vi "configureAnalogOutput.vi"(8 "error in (no error)":errorcluster, 9 "AnalogOutput":refnum<class "AnalogOutput.lvclass">, 10 "deviceName":string, 11 "AtomChipHWC in":refnum<class "AtomChipHWC.lvclass">) -> (0 "error out":errorcluster, 3 "AtomChipHWC out":refnum<class "AtomChipHWC.lvclass">)   [LabVIEW 2011, in "Hardware.lvlib" / "HWControllers.lvlib" / "AtomChipHWC.lvclass"]
doc: "Configure the analog channels of a device"
uses:
  AtomChipHWC.lvclass
  Channels/VoltOutput/AnalogOutput.lvclass
  AtomChipHWC.lvclass/AtomChipHWC.ctl
  HWController.lvclass
  Tools/Filing/FileNeologist/FileNeologist.lvclass
  Tools/Filing.lvlib
  Tools/DatabaseHelpers/DbConnection/DeviceDataBase/deviceDataBase.lvclass
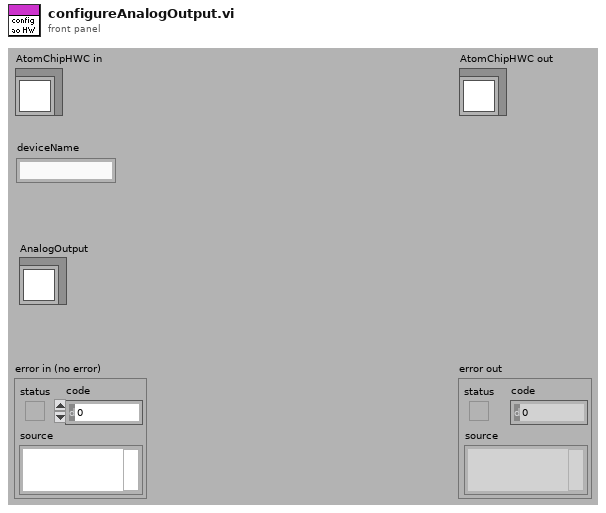
[diagram p1: front panel]
types:
  T1 = cluster{string, "Physical Channels":string, "Ranges":dbl[]}
  T2 = cluster{"Clock source":string, "Clock rate":dbl, "Start trigger line":string, "Sample Rate":dbl, "Sample No.":dbl}
  T3 = cluster{"Range":cluster{"current":dbl, "voltage":dbl}, "triggering_inUse":cluster{"start_trigger":string, "clock":string}, "Limits":cluster{"VoltageLimit":dbl, "CurrentLimit":dbl}}[]
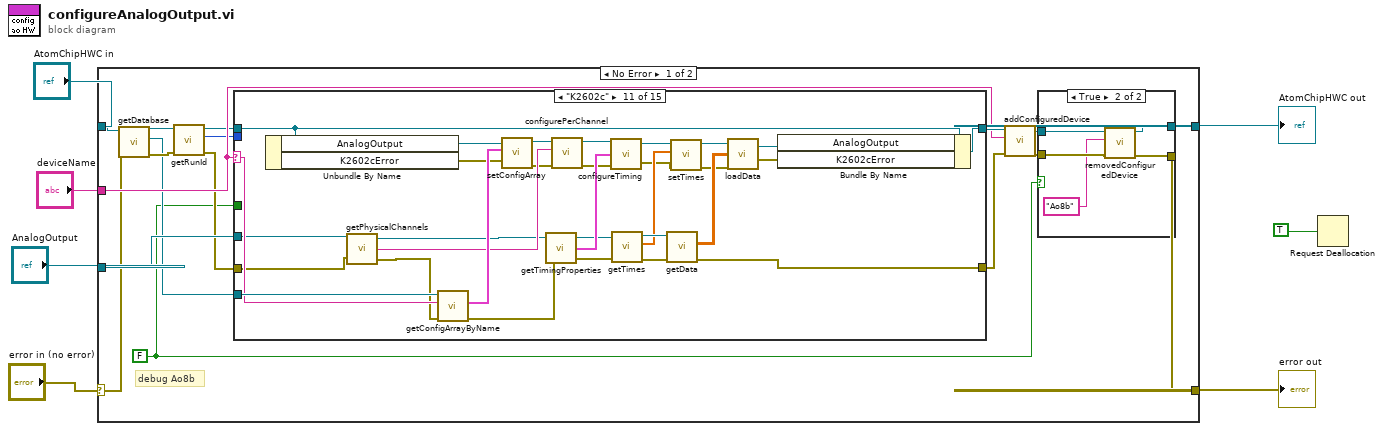
[diagram p0: block diagram]
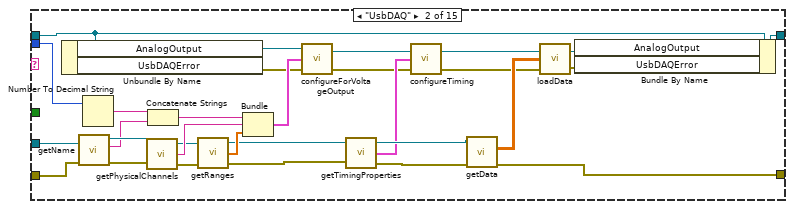
[diagram p4: hidden frame]
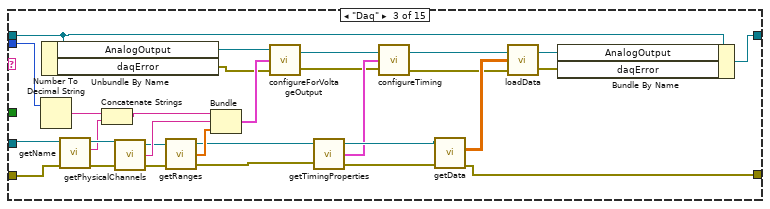
[diagram p5: hidden frame]
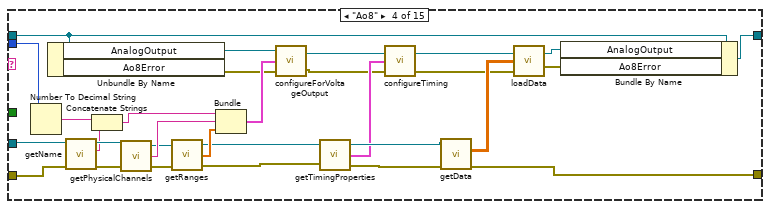
[diagram p6: hidden frame]
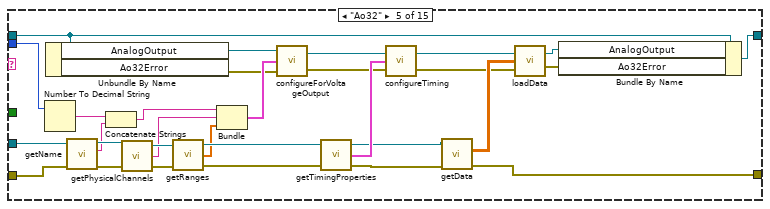
[diagram p7: hidden frame]
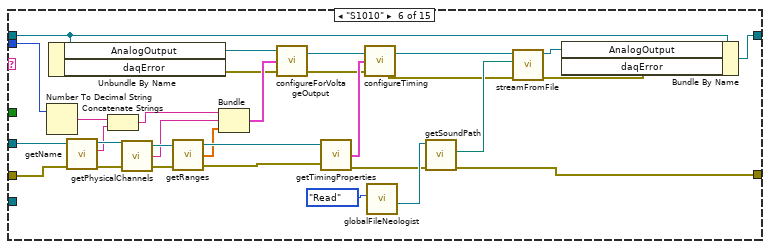
[diagram p8: hidden frame]
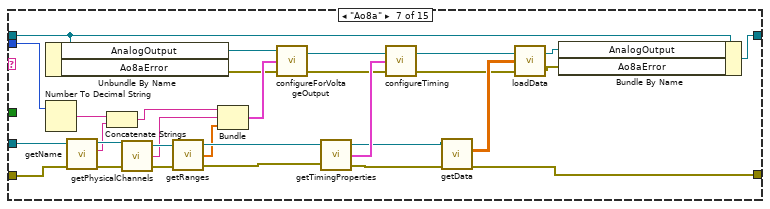
[diagram p9: hidden frame]
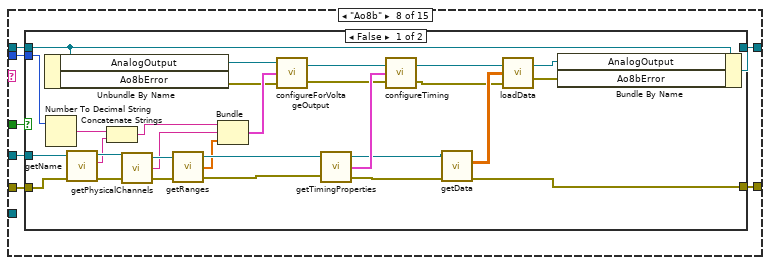
[diagram p10: hidden frame]
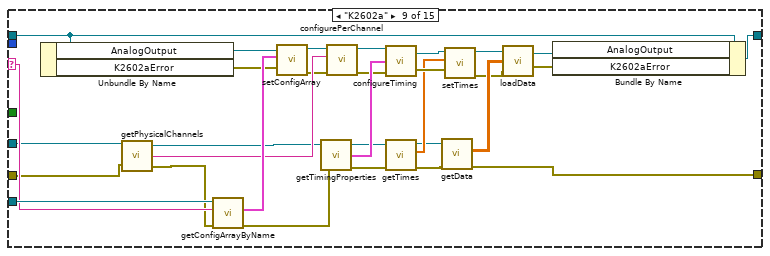
[diagram p12: hidden frame]
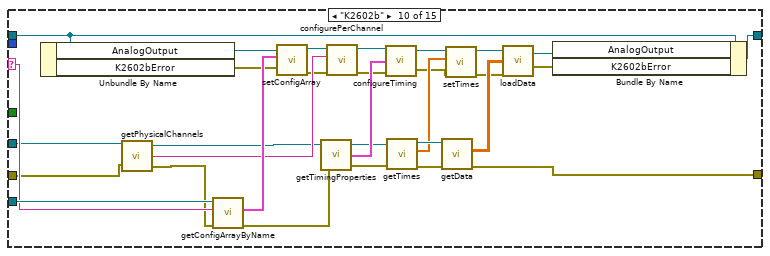
[diagram p13: hidden frame]
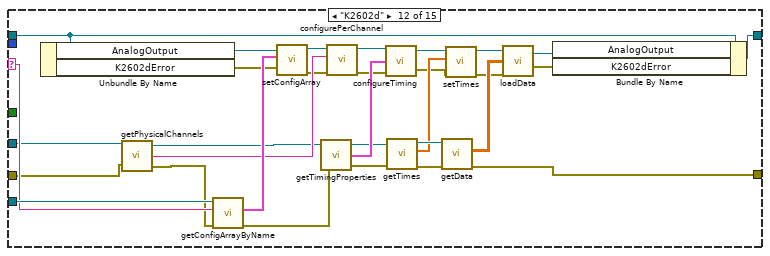
[diagram p14: hidden frame]
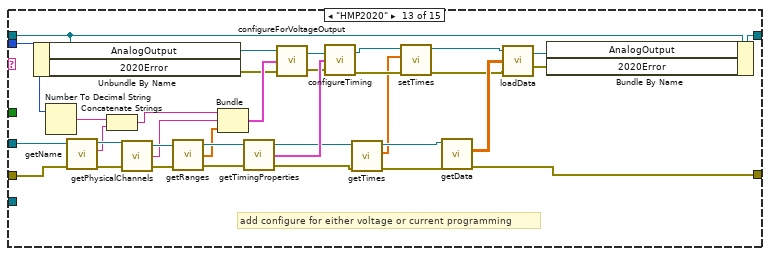
[diagram p15: hidden frame]
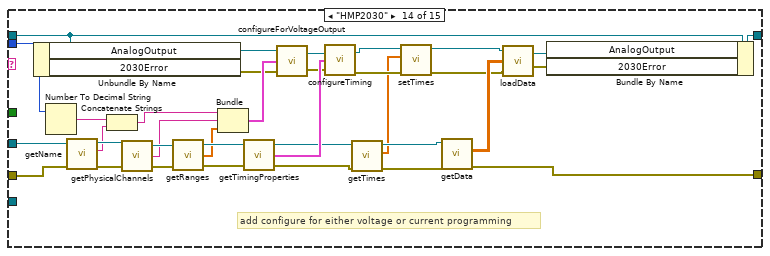
[diagram p16: hidden frame]
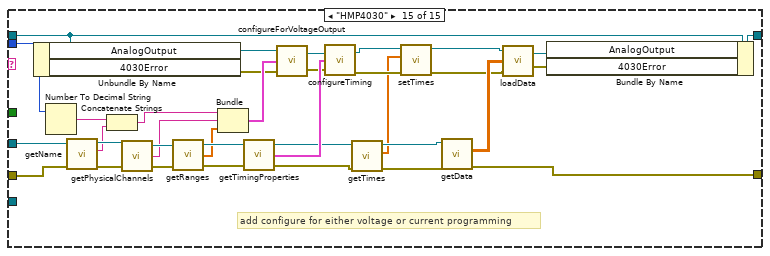
[diagram p17: hidden frame]
diagram:
  n1 = case shown="No Error" "error in (no error)" {
    selector: "error in (no error)" -> [w15 w484]
    tunnel: [w9 w484] -> w6
    tunnel: [w11 w483] -> w4
    tunnel: "AtomChipHWC in" -> [w16 w483]
    tunnel: "deviceName" -> [w21 _]
    tunnel: "AnalogOutput" -> [w24 _]
    frame No Error {
      w8 = FALSE
      # "debug Ao8b"
      n2 = call "getDatabase.vi"("error in (no error)"=w15, "HWController in"=w16) -> ("error out"=w14:errorcluster, "deviceDataBase"=w13:refnum<class "deviceDataBase.lvclass">, "HWController out"=w17:refnum<class "AtomChipHWC.lvclass">)  [unwired: 7 in]
      n3 = call "getRunId.vi"("error in (no error)"=w14, "HWController in"=w17) -> ("error out"=w19:errorcluster, "Numeric"=w18:i32, "HWController out"=w20:refnum<class "AtomChipHWC.lvclass">)  [unwired: 7 in]
      n4 = case shown="\"K2602c\"" w21 {
        selector: w21 -> [_ _ _ _ _ _ _ _ w276 w307 w338 w369 _ _ _]
        tunnel: w20 -> [w33 w48 w78 w108 w153 w184 w214 w221 w284 w315 w346 w377 w412 w447 w482]
        tunnel: [w33 w47 w77 w107 w152 w183 w213 w220 w283 w314 w345 w376 w411 w446 w481] -> w23
        tunnel: [w32 w34 w65 w95 w126 w156 w185 w216 w278 w309 w340 w371 w388 w423 w458] -> w22
        tunnel: w24 -> [_ w46 w76 w106 w145 w176 w206 w218 w270 w301 w332 w363 w404 w439 w474]
        tunnel: w19 -> [w32 w45 w75 w105 w146 w177 w207 w219 w269 w300 w331 w362 w405 w440 w475]
        tunnel: w18 -> [_ w41 w73 w103 w133 w168 w194 w217 _ _ _ _ w394 w429 w464]
        tunnel: w13 -> [_ _ _ _ _ _ _ _ w277 w308 w339 w370 _ _ _]
        tunnel: w8 -> [_ _ _ _ _ _ _ w215 _ _ _ _ _ _ _]
        frame "No Hardware", Default {
        }
        frame "UsbDAQ" {
          n5 = Unbundle By Name(w48) -> ("AnalogOutput"=w54:refnum<class "AnalogOutput.lvclass">, "UsbDAQError"=w37:errorcluster)
          n6 = call "getName.vi"("error in (no error)"=w45, "AnalogOutput.lvclass in"=w46) -> ("error out"=w49:errorcluster, "name"=w43:string, "AnalogOutput.lvclass out"=w51:refnum<class "AnalogOutput.lvclass">)  [unwired: 7 in]
          n7 = Number To Decimal String(number=w41) -> (decimal integer string=w44:string)  [unwired: 1 in]
          n8 = call-dynamic "getPhysicalChannels.vi"("AnalogOutput.lvclass in"=w51, "error in (no error)"=w49) -> ("AnalogOutput.lvclass out"=w52:refnum<class "AnalogOutput.lvclass">, "Physical Channels"=w55:string, "error out"=w50:errorcluster)
          n9 = Concatenate Strings(w44, w43) -> (w42:string)
          n10 = call "getRanges.vi"("AnalogOutput.lvclass in"=w52, "error in (no error)"=w50) -> ("AnalogOutput.lvclass out"=w53:refnum<class "AnalogOutput.lvclass">, "Ranges"=w56:dbl[], "error out"=w36:errorcluster)
          n11 = Bundle(w42, "Physical Channels"=w55, "Ranges"=w56) -> (w57:T1)  [unwired: 1 in]
          n12 = call-dynamic "configureForVoltageOutput.vi"("error in (no error)"=w37, "Output Properties"=w57, "AnalogOutput in"=w54) -> ("error out"=w38:errorcluster, "AnalogOutput out"=w60:refnum<class "AnalogOutput.lvclass">)
          n13 = call "getTimingProperties.vi"("AnalogOutput.lvclass in"=w53, "error in (no error)"=w36) -> ("AnalogOutput.lvclass out"=w59:refnum<class "AnalogOutput.lvclass">, "Timing"=w58:T2, "error out"=w35:errorcluster)
          n14 = call-dynamic "configureTiming.vi"("error in (no error)"=w38, "Timing"=w58, "AnalogOutput in"=w60) -> ("error out"=w39:errorcluster, "AnalogOutput out"=w61:refnum<class "AnalogOutput.lvclass">)
          n15 = call "getData.vi"("error in (no error)"=w35, "AnalogOutput.lvclass in"=w59) -> ("error out"=w34:errorcluster, "Data"=w62:dbl[][])  [unwired: 7 in, 1 out]
          n16 = call-dynamic "loadData.vi"("error in (no error)"=w39, "Data"=w62, "AnalogOutput in"=w61) -> ("error out"=w40:errorcluster, "AnalogOutput out"=w63:refnum<class "AnalogOutput.lvclass">)
          n17 = Bundle By Name(cluster=w48, "AnalogOutput"=w63, "UsbDAQError"=w40) -> (w47:refnum<class "AtomChipHWC.lvclass">)
        }
        frame "Daq" {
          n18 = Number To Decimal String(number=w73) -> (decimal integer string=w74:string)  [unwired: 1 in]
          n19 = Unbundle By Name(w78) -> ("AnalogOutput"=w84:refnum<class "AnalogOutput.lvclass">, "daqError"=w68:errorcluster)
          n20 = call "getName.vi"("error in (no error)"=w75, "AnalogOutput.lvclass in"=w76) -> ("error out"=w79:errorcluster, "name"=w72:string, "AnalogOutput.lvclass out"=w81:refnum<class "AnalogOutput.lvclass">)  [unwired: 7 in]
          n21 = Concatenate Strings(w74, w72) -> (w71:string)
          n22 = call-dynamic "getPhysicalChannels.vi"("AnalogOutput.lvclass in"=w81, "error in (no error)"=w79) -> ("AnalogOutput.lvclass out"=w82:refnum<class "AnalogOutput.lvclass">, "Physical Channels"=w85:string, "error out"=w80:errorcluster)
          n23 = call "getRanges.vi"("AnalogOutput.lvclass in"=w82, "error in (no error)"=w80) -> ("AnalogOutput.lvclass out"=w83:refnum<class "AnalogOutput.lvclass">, "Ranges"=w86:dbl[], "error out"=w70:errorcluster)
          n24 = Bundle(w71, "Physical Channels"=w85, "Ranges"=w86) -> (w87:T1)  [unwired: 1 in]
          n25 = call-dynamic "configureForVoltageOutput.vi"("error in (no error)"=w68, "Output Properties"=w87, "AnalogOutput in"=w84) -> ("error out"=w66:errorcluster, "AnalogOutput out"=w90:refnum<class "AnalogOutput.lvclass">)
          n26 = call "getTimingProperties.vi"("AnalogOutput.lvclass in"=w83, "error in (no error)"=w70) -> ("AnalogOutput.lvclass out"=w89:refnum<class "AnalogOutput.lvclass">, "Timing"=w88:T2, "error out"=w67:errorcluster)
          n27 = call-dynamic "configureTiming.vi"("error in (no error)"=w66, "Timing"=w88, "AnalogOutput in"=w90) -> ("error out"=w69:errorcluster, "AnalogOutput out"=w91:refnum<class "AnalogOutput.lvclass">)
          n28 = call "getData.vi"("error in (no error)"=w67, "AnalogOutput.lvclass in"=w89) -> ("error out"=w65:errorcluster, "Data"=w92:dbl[][])  [unwired: 7 in, 1 out]
          n29 = call-dynamic "loadData.vi"("error in (no error)"=w69, "Data"=w92, "AnalogOutput in"=w91) -> ("error out"=w64:errorcluster, "AnalogOutput out"=w93:refnum<class "AnalogOutput.lvclass">)
          n30 = Bundle By Name(cluster=w78, "AnalogOutput"=w93, "daqError"=w64) -> (w77:refnum<class "AtomChipHWC.lvclass">)
        }
        frame "Ao8" {
          n31 = Number To Decimal String(number=w103) -> (decimal integer string=w104:string)  [unwired: 1 in]
          n32 = Unbundle By Name(w108) -> ("AnalogOutput"=w114:refnum<class "AnalogOutput.lvclass">, "Ao8Error"=w98:errorcluster)
          n33 = call "getName.vi"("error in (no error)"=w105, "AnalogOutput.lvclass in"=w106) -> ("error out"=w109:errorcluster, "name"=w102:string, "AnalogOutput.lvclass out"=w111:refnum<class "AnalogOutput.lvclass">)  [unwired: 7 in]
          n34 = Concatenate Strings(w104, w102) -> (w101:string)
          n35 = call-dynamic "getPhysicalChannels.vi"("AnalogOutput.lvclass in"=w111, "error in (no error)"=w109) -> ("AnalogOutput.lvclass out"=w112:refnum<class "AnalogOutput.lvclass">, "Physical Channels"=w115:string, "error out"=w110:errorcluster)
          n36 = call "getRanges.vi"("AnalogOutput.lvclass in"=w112, "error in (no error)"=w110) -> ("AnalogOutput.lvclass out"=w113:refnum<class "AnalogOutput.lvclass">, "Ranges"=w116:dbl[], "error out"=w97:errorcluster)
          n37 = Bundle(w101, "Physical Channels"=w115, "Ranges"=w116) -> (w117:T1)  [unwired: 1 in]
          n38 = call-dynamic "configureForVoltageOutput.vi"("error in (no error)"=w98, "Output Properties"=w117, "AnalogOutput in"=w114) -> ("error out"=w99:errorcluster, "AnalogOutput out"=w120:refnum<class "AnalogOutput.lvclass">)
          n39 = call "getTimingProperties.vi"("AnalogOutput.lvclass in"=w113, "error in (no error)"=w97) -> ("AnalogOutput.lvclass out"=w119:refnum<class "AnalogOutput.lvclass">, "Timing"=w118:T2, "error out"=w96:errorcluster)
          n40 = call-dynamic "configureTiming.vi"("error in (no error)"=w99, "Timing"=w118, "AnalogOutput in"=w120) -> ("error out"=w100:errorcluster, "AnalogOutput out"=w121:refnum<class "AnalogOutput.lvclass">)
          n41 = call "getData.vi"("error in (no error)"=w96, "AnalogOutput.lvclass in"=w119) -> ("error out"=w95:errorcluster, "Data"=w122:dbl[][])  [unwired: 7 in, 1 out]
          n42 = call-dynamic "loadData.vi"("error in (no error)"=w100, "Data"=w122, "AnalogOutput in"=w121) -> ("error out"=w94:errorcluster, "AnalogOutput out"=w123:refnum<class "AnalogOutput.lvclass">)
          n43 = Bundle By Name(cluster=w108, "AnalogOutput"=w123, "Ao8Error"=w94) -> (w107:refnum<class "AtomChipHWC.lvclass">)
        }
        frame "Ao32" {
          n44 = Number To Decimal String(number=w133) -> (decimal integer string=w134:string)  [unwired: 1 in]
          n45 = Unbundle By Name(w153) -> ("AnalogOutput"=w144:refnum<class "AnalogOutput.lvclass">, "Ao32Error"=w130:errorcluster)
          n46 = call "getName.vi"("error in (no error)"=w146, "AnalogOutput.lvclass in"=w145) -> ("error out"=w151:errorcluster, "name"=w132:string, "AnalogOutput.lvclass out"=w149:refnum<class "AnalogOutput.lvclass">)  [unwired: 7 in]
          n47 = Concatenate Strings(w134, w132) -> (w131:string)
          n48 = call-dynamic "getPhysicalChannels.vi"("AnalogOutput.lvclass in"=w149, "error in (no error)"=w151) -> ("AnalogOutput.lvclass out"=w148:refnum<class "AnalogOutput.lvclass">, "Physical Channels"=w143:string, "error out"=w150:errorcluster)
          n49 = call "getRanges.vi"("AnalogOutput.lvclass in"=w148, "error in (no error)"=w150) -> ("AnalogOutput.lvclass out"=w147:refnum<class "AnalogOutput.lvclass">, "Ranges"=w142:dbl[], "error out"=w124:errorcluster)
          n50 = Bundle(w131, "Physical Channels"=w143, "Ranges"=w142) -> (w141:T1)  [unwired: 1 in]
          n51 = call-dynamic "configureForVoltageOutput.vi"("error in (no error)"=w130, "Output Properties"=w141, "AnalogOutput in"=w144) -> ("error out"=w129:errorcluster, "AnalogOutput out"=w138:refnum<class "AnalogOutput.lvclass">)
          n52 = call "getTimingProperties.vi"("AnalogOutput.lvclass in"=w147, "error in (no error)"=w124) -> ("AnalogOutput.lvclass out"=w139:refnum<class "AnalogOutput.lvclass">, "Timing"=w140:T2, "error out"=w125:errorcluster)
          n53 = call-dynamic "configureTiming.vi"("error in (no error)"=w129, "Timing"=w140, "AnalogOutput in"=w138) -> ("error out"=w128:errorcluster, "AnalogOutput out"=w137:refnum<class "AnalogOutput.lvclass">)
          n54 = call "getData.vi"("error in (no error)"=w125, "AnalogOutput.lvclass in"=w139) -> ("error out"=w126:errorcluster, "Data"=w136:dbl[][])  [unwired: 7 in, 1 out]
          n55 = call-dynamic "loadData.vi"("error in (no error)"=w128, "Data"=w136, "AnalogOutput in"=w137) -> ("error out"=w127:errorcluster, "AnalogOutput out"=w135:refnum<class "AnalogOutput.lvclass">)
          n56 = Bundle By Name(cluster=w153, "AnalogOutput"=w135, "Ao32Error"=w127) -> (w152:refnum<class "AtomChipHWC.lvclass">)
        }
        frame "S1010" {
          n57 = Number To Decimal String(number=w168) -> (decimal integer string=w169:string)  [unwired: 1 in]
          n58 = Unbundle By Name(w184) -> ("AnalogOutput"=w175:refnum<class "AnalogOutput.lvclass">, "daqError"=w158:errorcluster)
          n59 = call "getName.vi"("error in (no error)"=w177, "AnalogOutput.lvclass in"=w176) -> ("error out"=w182:errorcluster, "name"=w167:string, "AnalogOutput.lvclass out"=w180:refnum<class "AnalogOutput.lvclass">)  [unwired: 7 in]
          n60 = Concatenate Strings(w169, w167) -> (w166:string)
          n61 = call-dynamic "getPhysicalChannels.vi"("AnalogOutput.lvclass in"=w180, "error in (no error)"=w182) -> ("AnalogOutput.lvclass out"=w179:refnum<class "AnalogOutput.lvclass">, "Physical Channels"=w174:string, "error out"=w181:errorcluster)
          n62 = call "getRanges.vi"("AnalogOutput.lvclass in"=w179, "error in (no error)"=w181) -> ("AnalogOutput.lvclass out"=w178:refnum<class "AnalogOutput.lvclass">, "Ranges"=w173:dbl[], "error out"=w154:errorcluster)
          n63 = Bundle(w166, "Physical Channels"=w174, "Ranges"=w173) -> (w172:T1)  [unwired: 1 in]
          n64 = call-dynamic "configureForVoltageOutput.vi"("error in (no error)"=w158, "Output Properties"=w172, "AnalogOutput in"=w175) -> ("error out"=w159:errorcluster, "AnalogOutput out"=w170:refnum<class "AnalogOutput.lvclass">)
          n65 = call "getTimingProperties.vi"("AnalogOutput.lvclass in"=w178, "error in (no error)"=w154) -> ("Timing"=w171:T2, "error out"=w155:errorcluster)  [unwired: 1 out]
          n66 = call-dynamic "configureTiming.vi"("error in (no error)"=w159, "Timing"=w171, "AnalogOutput in"=w170) -> ("error out"=w160:errorcluster, "AnalogOutput out"=w165:refnum<class "AnalogOutput.lvclass">)
          n67 = call "globalFileNeologist.vi"("Action"=enum16{"Write", "Read"}."Read") -> ("FileNeologist out"=w163:refnum<class "FileNeologist.lvclass">)  [unwired: 10 in]
          n68 = call "getSoundPath.vi"("error in (no error)"=w155, "FileNeologist in"=w163) -> ("error out"=w156:errorcluster, "Path"=w161:path)  [unwired: 7 in, 1 out]
          n69 = call-dynamic "streamFromFile.vi"("error in (no error)"=w160, "Path"=w161, "AnalogOutput in"=w165) -> ("error out"=w157:errorcluster, "AnalogOutput out"=w164:refnum<class "AnalogOutput.lvclass">)  [unwired: 7 in]
          n70 = Bundle By Name(cluster=w184, "AnalogOutput"=w164, "daqError"=w157) -> (w183:refnum<class "AtomChipHWC.lvclass">)
        }
        frame "Ao8a" {
          n71 = Unbundle By Name(w214) -> ("AnalogOutput"=w205:refnum<class "AnalogOutput.lvclass">, "Ao8aError"=w189:errorcluster)
          n72 = Number To Decimal String(number=w194) -> (decimal integer string=w195:string)  [unwired: 1 in]
          n73 = call "getName.vi"("error in (no error)"=w207, "AnalogOutput.lvclass in"=w206) -> ("error out"=w212:errorcluster, "name"=w193:string, "AnalogOutput.lvclass out"=w210:refnum<class "AnalogOutput.lvclass">)  [unwired: 7 in]
          n74 = Concatenate Strings(w195, w193) -> (w192:string)
          n75 = call-dynamic "getPhysicalChannels.vi"("AnalogOutput.lvclass in"=w210, "error in (no error)"=w212) -> ("AnalogOutput.lvclass out"=w209:refnum<class "AnalogOutput.lvclass">, "Physical Channels"=w204:string, "error out"=w211:errorcluster)
          n76 = call "getRanges.vi"("AnalogOutput.lvclass in"=w209, "error in (no error)"=w211) -> ("AnalogOutput.lvclass out"=w208:refnum<class "AnalogOutput.lvclass">, "Ranges"=w203:dbl[], "error out"=w186:errorcluster)
          n77 = Bundle(w192, "Physical Channels"=w204, "Ranges"=w203) -> (w202:T1)  [unwired: 1 in]
          n78 = call-dynamic "configureForVoltageOutput.vi"("error in (no error)"=w189, "Output Properties"=w202, "AnalogOutput in"=w205) -> ("error out"=w190:errorcluster, "AnalogOutput out"=w199:refnum<class "AnalogOutput.lvclass">)
          n79 = call "getTimingProperties.vi"("AnalogOutput.lvclass in"=w208, "error in (no error)"=w186) -> ("AnalogOutput.lvclass out"=w200:refnum<class "AnalogOutput.lvclass">, "Timing"=w201:T2, "error out"=w187:errorcluster)
          n80 = call-dynamic "configureTiming.vi"("error in (no error)"=w190, "Timing"=w201, "AnalogOutput in"=w199) -> ("error out"=w191:errorcluster, "AnalogOutput out"=w198:refnum<class "AnalogOutput.lvclass">)
          n81 = call "getData.vi"("error in (no error)"=w187, "AnalogOutput.lvclass in"=w200) -> ("error out"=w185:errorcluster, "Data"=w197:dbl[][])  [unwired: 7 in, 1 out]
          n82 = call-dynamic "loadData.vi"("error in (no error)"=w191, "Data"=w197, "AnalogOutput in"=w198) -> ("error out"=w188:errorcluster, "AnalogOutput out"=w196:refnum<class "AnalogOutput.lvclass">)
          n83 = Bundle By Name(cluster=w214, "AnalogOutput"=w196, "Ao8aError"=w188) -> (w213:refnum<class "AtomChipHWC.lvclass">)
        }
        frame "Ao8b" {
          n84 = case shown="False" w215 {
            tunnel: w221 -> [w251 w253]
            tunnel: [w250 w253] -> w220
            tunnel: w219 -> [w249 w252]
            tunnel: w218 -> [w248 _]
            tunnel: w217 -> [w247 _]
            tunnel: [w246 w252] -> w216
            frame False {
              n85 = Unbundle By Name(w251) -> ("AnalogOutput"=w240:refnum<class "AnalogOutput.lvclass">, "Ao8bError"=w227:errorcluster)
              n86 = Number To Decimal String(number=w247) -> (decimal integer string=w230:string)  [unwired: 1 in]
              n87 = call "getName.vi"("error in (no error)"=w249, "AnalogOutput.lvclass in"=w248) -> ("error out"=w245:errorcluster, "name"=w229:string, "AnalogOutput.lvclass out"=w243:refnum<class "AnalogOutput.lvclass">)  [unwired: 7 in]
              n88 = Concatenate Strings(w230, w229) -> (w228:string)
              n89 = call-dynamic "getPhysicalChannels.vi"("AnalogOutput.lvclass in"=w243, "error in (no error)"=w245) -> ("AnalogOutput.lvclass out"=w242:refnum<class "AnalogOutput.lvclass">, "Physical Channels"=w239:string, "error out"=w244:errorcluster)
              n90 = call "getRanges.vi"("AnalogOutput.lvclass in"=w242, "error in (no error)"=w244) -> ("AnalogOutput.lvclass out"=w241:refnum<class "AnalogOutput.lvclass">, "Ranges"=w238:dbl[], "error out"=w222:errorcluster)
              n91 = Bundle(w228, "Physical Channels"=w239, "Ranges"=w238) -> (w237:T1)  [unwired: 1 in]
              n92 = call-dynamic "configureForVoltageOutput.vi"("error in (no error)"=w227, "Output Properties"=w237, "AnalogOutput in"=w240) -> ("error out"=w226:errorcluster, "AnalogOutput out"=w234:refnum<class "AnalogOutput.lvclass">)
              n93 = call "getTimingProperties.vi"("AnalogOutput.lvclass in"=w241, "error in (no error)"=w222) -> ("AnalogOutput.lvclass out"=w235:refnum<class "AnalogOutput.lvclass">, "Timing"=w236:T2, "error out"=w223:errorcluster)
              n94 = call-dynamic "configureTiming.vi"("error in (no error)"=w226, "Timing"=w236, "AnalogOutput in"=w234) -> ("error out"=w225:errorcluster, "AnalogOutput out"=w233:refnum<class "AnalogOutput.lvclass">)
              n95 = call "getData.vi"("error in (no error)"=w223, "AnalogOutput.lvclass in"=w235) -> ("error out"=w246:errorcluster, "Data"=w232:dbl[][])  [unwired: 7 in, 1 out]
              n96 = call-dynamic "loadData.vi"("error in (no error)"=w225, "Data"=w232, "AnalogOutput in"=w233) -> ("error out"=w224:errorcluster, "AnalogOutput out"=w231:refnum<class "AnalogOutput.lvclass">)
              n97 = Bundle By Name(cluster=w251, "AnalogOutput"=w231, "Ao8bError"=w224) -> (w250:refnum<class "AtomChipHWC.lvclass">)
            }
            frame True {
            }
          }
        }
        frame "K2602a" {
          n98 = Unbundle By Name(w284) -> ("AnalogOutput"=w266:refnum<class "AnalogOutput.lvclass">, "K2602aError"=w263:errorcluster)
          n99 = call-dynamic "getPhysicalChannels.vi"("AnalogOutput.lvclass in"=w270, "error in (no error)"=w269) -> ("AnalogOutput.lvclass out"=w272:refnum<class "AnalogOutput.lvclass">, "Physical Channels"=w273:string, "error out"=w271:errorcluster)
          n100 = call "getConfigArrayByName.vi"("error in (no error)"=w271, "device_name"=w276, "deviceDataBase in"=w277) -> ("error out"=w275:errorcluster, "ConfigArray"=w274:T3)  [unwired: 6 in, 1 out]
          n101 = call-dynamic "setConfigArray.vi"("error in (no error)"=w263, "ConfigArray"=w274, "AnalogOutput in"=w266) -> ("error out"=w264:errorcluster, "AnalogOutput out"=w265:refnum<class "AnalogOutput.lvclass">)  [unwired: 7 in]
          n102 = call "getTimingProperties.vi"("AnalogOutput.lvclass in"=w272, "error in (no error)"=w275) -> ("AnalogOutput.lvclass out"=w258:refnum<class "AnalogOutput.lvclass">, "Timing"=w282:T2, "error out"=w257:errorcluster)
          n103 = call-dynamic "configurePerChannel.vi"("error in (no error)"=w264, "physical channels"=w273, "AnalogOutput in"=w265) -> ("error out"=w267:errorcluster, "AnalogOutput out"=w268:refnum<class "AnalogOutput.lvclass">)  [unwired: 7 in]
          n104 = call-dynamic "configureTiming.vi"("error in (no error)"=w267, "Timing"=w282, "AnalogOutput in"=w268) -> ("error out"=w261:errorcluster, "AnalogOutput out"=w262:refnum<class "AnalogOutput.lvclass">)
          n105 = call "getTimes.vi"("error in (no error)"=w257, "AnalogOutput in"=w258) -> ("error out"=w256:errorcluster, "times"=w255:dbl[], "AnalogOutput out"=w254:refnum<class "AnalogOutput.lvclass">)  [unwired: 7 in]
          n106 = call "getData.vi"("error in (no error)"=w256, "AnalogOutput.lvclass in"=w254) -> ("error out"=w278:errorcluster, "Data"=w281:dbl[][])  [unwired: 7 in, 1 out]
          n107 = call "setTimes.vi"("error in (no error)"=w261, "times"=w255, "AnalogOutput in"=w262) -> ("error out"=w260:errorcluster, "AnalogOutput out"=w259:refnum<class "AnalogOutput.lvclass">)  [unwired: 7 in]
          n108 = call-dynamic "loadData.vi"("error in (no error)"=w260, "Data"=w281, "AnalogOutput in"=w259) -> ("error out"=w279:errorcluster, "AnalogOutput out"=w280:refnum<class "AnalogOutput.lvclass">)
          n109 = Bundle By Name(cluster=w284, "AnalogOutput"=w280, "K2602aError"=w279) -> (w283:refnum<class "AtomChipHWC.lvclass">)
        }
        frame "K2602b" {
          n110 = Unbundle By Name(w315) -> ("AnalogOutput"=w297:refnum<class "AnalogOutput.lvclass">, "K2602bError"=w294:errorcluster)
          n111 = call-dynamic "getPhysicalChannels.vi"("AnalogOutput.lvclass in"=w301, "error in (no error)"=w300) -> ("AnalogOutput.lvclass out"=w303:refnum<class "AnalogOutput.lvclass">, "Physical Channels"=w304:string, "error out"=w302:errorcluster)
          n112 = call "getConfigArrayByName.vi"("error in (no error)"=w302, "device_name"=w307, "deviceDataBase in"=w308) -> ("error out"=w306:errorcluster, "ConfigArray"=w305:T3)  [unwired: 6 in, 1 out]
          n113 = call-dynamic "setConfigArray.vi"("error in (no error)"=w294, "ConfigArray"=w305, "AnalogOutput in"=w297) -> ("error out"=w295:errorcluster, "AnalogOutput out"=w296:refnum<class "AnalogOutput.lvclass">)  [unwired: 7 in]
          n114 = call "getTimingProperties.vi"("AnalogOutput.lvclass in"=w303, "error in (no error)"=w306) -> ("AnalogOutput.lvclass out"=w293:refnum<class "AnalogOutput.lvclass">, "Timing"=w313:T2, "error out"=w285:errorcluster)
          n115 = call-dynamic "configurePerChannel.vi"("error in (no error)"=w295, "physical channels"=w304, "AnalogOutput in"=w296) -> ("error out"=w298:errorcluster, "AnalogOutput out"=w299:refnum<class "AnalogOutput.lvclass">)  [unwired: 7 in]
          n116 = call-dynamic "configureTiming.vi"("error in (no error)"=w298, "Timing"=w313, "AnalogOutput in"=w299) -> ("error out"=w289:errorcluster, "AnalogOutput out"=w290:refnum<class "AnalogOutput.lvclass">)
          n117 = call "getTimes.vi"("error in (no error)"=w285, "AnalogOutput in"=w293) -> ("error out"=w286:errorcluster, "times"=w291:dbl[], "AnalogOutput out"=w292:refnum<class "AnalogOutput.lvclass">)  [unwired: 7 in]
          n118 = call "getData.vi"("error in (no error)"=w286, "AnalogOutput.lvclass in"=w292) -> ("error out"=w309:errorcluster, "Data"=w312:dbl[][])  [unwired: 7 in, 1 out]
          n119 = call "setTimes.vi"("error in (no error)"=w289, "times"=w291, "AnalogOutput in"=w290) -> ("error out"=w288:errorcluster, "AnalogOutput out"=w287:refnum<class "AnalogOutput.lvclass">)  [unwired: 7 in]
          n120 = call-dynamic "loadData.vi"("error in (no error)"=w288, "Data"=w312, "AnalogOutput in"=w287) -> ("error out"=w310:errorcluster, "AnalogOutput out"=w311:refnum<class "AnalogOutput.lvclass">)
          n121 = Bundle By Name(cluster=w315, "AnalogOutput"=w311, "K2602bError"=w310) -> (w314:refnum<class "AtomChipHWC.lvclass">)
        }
        frame "K2602c" {
          n122 = Unbundle By Name(w346) -> ("AnalogOutput"=w328:refnum<class "AnalogOutput.lvclass">, "K2602cError"=w325:errorcluster)
          n123 = call-dynamic "getPhysicalChannels.vi"("AnalogOutput.lvclass in"=w332, "error in (no error)"=w331) -> ("AnalogOutput.lvclass out"=w334:refnum<class "AnalogOutput.lvclass">, "Physical Channels"=w335:string, "error out"=w333:errorcluster)
          n124 = call "getConfigArrayByName.vi"("error in (no error)"=w333, "device_name"=w338, "deviceDataBase in"=w339) -> ("error out"=w337:errorcluster, "ConfigArray"=w336:T3)  [unwired: 6 in, 1 out]
          n125 = call-dynamic "setConfigArray.vi"("error in (no error)"=w325, "ConfigArray"=w336, "AnalogOutput in"=w328) -> ("error out"=w326:errorcluster, "AnalogOutput out"=w327:refnum<class "AnalogOutput.lvclass">)  [unwired: 7 in]
          n126 = call "getTimingProperties.vi"("AnalogOutput.lvclass in"=w334, "error in (no error)"=w337) -> ("AnalogOutput.lvclass out"=w324:refnum<class "AnalogOutput.lvclass">, "Timing"=w344:T2, "error out"=w316:errorcluster)
          n127 = call-dynamic "configurePerChannel.vi"("error in (no error)"=w326, "physical channels"=w335, "AnalogOutput in"=w327) -> ("error out"=w329:errorcluster, "AnalogOutput out"=w330:refnum<class "AnalogOutput.lvclass">)  [unwired: 7 in]
          n128 = call-dynamic "configureTiming.vi"("error in (no error)"=w329, "Timing"=w344, "AnalogOutput in"=w330) -> ("error out"=w320:errorcluster, "AnalogOutput out"=w321:refnum<class "AnalogOutput.lvclass">)
          n129 = call "getTimes.vi"("error in (no error)"=w316, "AnalogOutput in"=w324) -> ("error out"=w317:errorcluster, "times"=w322:dbl[], "AnalogOutput out"=w323:refnum<class "AnalogOutput.lvclass">)  [unwired: 7 in]
          n130 = call "getData.vi"("error in (no error)"=w317, "AnalogOutput.lvclass in"=w323) -> ("error out"=w340:errorcluster, "Data"=w343:dbl[][])  [unwired: 7 in, 1 out]
          n131 = call "setTimes.vi"("error in (no error)"=w320, "times"=w322, "AnalogOutput in"=w321) -> ("error out"=w319:errorcluster, "AnalogOutput out"=w318:refnum<class "AnalogOutput.lvclass">)  [unwired: 7 in]
          n132 = call-dynamic "loadData.vi"("error in (no error)"=w319, "Data"=w343, "AnalogOutput in"=w318) -> ("error out"=w341:errorcluster, "AnalogOutput out"=w342:refnum<class "AnalogOutput.lvclass">)
          n133 = Bundle By Name(cluster=w346, "AnalogOutput"=w342, "K2602cError"=w341) -> (w345:refnum<class "AtomChipHWC.lvclass">)
        }
        frame "K2602d" {
          n134 = Unbundle By Name(w377) -> ("AnalogOutput"=w359:refnum<class "AnalogOutput.lvclass">, "K2602dError"=w356:errorcluster)
          n135 = call-dynamic "getPhysicalChannels.vi"("AnalogOutput.lvclass in"=w363, "error in (no error)"=w362) -> ("AnalogOutput.lvclass out"=w365:refnum<class "AnalogOutput.lvclass">, "Physical Channels"=w366:string, "error out"=w364:errorcluster)
          n136 = call "getConfigArrayByName.vi"("error in (no error)"=w364, "device_name"=w369, "deviceDataBase in"=w370) -> ("error out"=w368:errorcluster, "ConfigArray"=w367:T3)  [unwired: 6 in, 1 out]
          n137 = call-dynamic "setConfigArray.vi"("error in (no error)"=w356, "ConfigArray"=w367, "AnalogOutput in"=w359) -> ("error out"=w357:errorcluster, "AnalogOutput out"=w358:refnum<class "AnalogOutput.lvclass">)  [unwired: 7 in]
          n138 = call "getTimingProperties.vi"("AnalogOutput.lvclass in"=w365, "error in (no error)"=w368) -> ("AnalogOutput.lvclass out"=w355:refnum<class "AnalogOutput.lvclass">, "Timing"=w375:T2, "error out"=w347:errorcluster)
          n139 = call-dynamic "configurePerChannel.vi"("error in (no error)"=w357, "physical channels"=w366, "AnalogOutput in"=w358) -> ("error out"=w360:errorcluster, "AnalogOutput out"=w361:refnum<class "AnalogOutput.lvclass">)  [unwired: 7 in]
          n140 = call-dynamic "configureTiming.vi"("error in (no error)"=w360, "Timing"=w375, "AnalogOutput in"=w361) -> ("error out"=w351:errorcluster, "AnalogOutput out"=w352:refnum<class "AnalogOutput.lvclass">)
          n141 = call "getTimes.vi"("error in (no error)"=w347, "AnalogOutput in"=w355) -> ("error out"=w348:errorcluster, "times"=w353:dbl[], "AnalogOutput out"=w354:refnum<class "AnalogOutput.lvclass">)  [unwired: 7 in]
          n142 = call "getData.vi"("error in (no error)"=w348, "AnalogOutput.lvclass in"=w354) -> ("error out"=w371:errorcluster, "Data"=w374:dbl[][])  [unwired: 7 in, 1 out]
          n143 = call "setTimes.vi"("error in (no error)"=w351, "times"=w353, "AnalogOutput in"=w352) -> ("error out"=w350:errorcluster, "AnalogOutput out"=w349:refnum<class "AnalogOutput.lvclass">)  [unwired: 7 in]
          n144 = call-dynamic "loadData.vi"("error in (no error)"=w350, "Data"=w374, "AnalogOutput in"=w349) -> ("error out"=w372:errorcluster, "AnalogOutput out"=w373:refnum<class "AnalogOutput.lvclass">)
          n145 = Bundle By Name(cluster=w377, "AnalogOutput"=w373, "K2602dError"=w372) -> (w376:refnum<class "AtomChipHWC.lvclass">)
        }
        frame "HMP2020" {
          # "add configure for either voltage or current programming"
          n146 = Unbundle By Name(w412) -> ("AnalogOutput"=w403:refnum<class "AnalogOutput.lvclass">, "2020Error"=w391:errorcluster)
          n147 = Number To Decimal String(number=w394) -> (decimal integer string=w395:string)  [unwired: 1 in]
          n148 = call "getName.vi"("error in (no error)"=w405, "AnalogOutput.lvclass in"=w404) -> ("error out"=w410:errorcluster, "name"=w393:string, "AnalogOutput.lvclass out"=w408:refnum<class "AnalogOutput.lvclass">)  [unwired: 7 in]
          n149 = Concatenate Strings(w395, w393) -> (w392:string)
          n150 = call-dynamic "getPhysicalChannels.vi"("AnalogOutput.lvclass in"=w408, "error in (no error)"=w410) -> ("AnalogOutput.lvclass out"=w407:refnum<class "AnalogOutput.lvclass">, "Physical Channels"=w402:string, "error out"=w409:errorcluster)
          n151 = call "getRanges.vi"("AnalogOutput.lvclass in"=w407, "error in (no error)"=w409) -> ("AnalogOutput.lvclass out"=w406:refnum<class "AnalogOutput.lvclass">, "Ranges"=w401:dbl[], "error out"=w387:errorcluster)
          n152 = Bundle(w392, "Physical Channels"=w402, "Ranges"=w401) -> (w400:T1)  [unwired: 1 in]
          n153 = call "getTimingProperties.vi"("AnalogOutput.lvclass in"=w406, "error in (no error)"=w387) -> ("AnalogOutput.lvclass out"=w386:refnum<class "AnalogOutput.lvclass">, "Timing"=w399:T2, "error out"=w385:errorcluster)
          n154 = call-dynamic "configureForVoltageOutput.vi"("error in (no error)"=w391, "Output Properties"=w400, "AnalogOutput in"=w403) -> ("error out"=w390:errorcluster, "AnalogOutput out"=w398:refnum<class "AnalogOutput.lvclass">)
          n155 = call-dynamic "configureTiming.vi"("error in (no error)"=w390, "Timing"=w399, "AnalogOutput in"=w398) -> ("error out"=w381:errorcluster, "AnalogOutput out"=w382:refnum<class "AnalogOutput.lvclass">)
          n156 = call "getTimes.vi"("error in (no error)"=w385, "AnalogOutput in"=w386) -> ("error out"=w383:errorcluster, "times"=w378:dbl[], "AnalogOutput out"=w384:refnum<class "AnalogOutput.lvclass">)  [unwired: 7 in]
          n157 = call "setTimes.vi"("error in (no error)"=w381, "times"=w378, "AnalogOutput in"=w382) -> ("error out"=w380:errorcluster, "AnalogOutput out"=w379:refnum<class "AnalogOutput.lvclass">)  [unwired: 7 in]
          n158 = call "getData.vi"("error in (no error)"=w383, "AnalogOutput.lvclass in"=w384) -> ("error out"=w388:errorcluster, "Data"=w397:dbl[][])  [unwired: 7 in, 1 out]
          n159 = call-dynamic "loadData.vi"("error in (no error)"=w380, "Data"=w397, "AnalogOutput in"=w379) -> ("error out"=w389:errorcluster, "AnalogOutput out"=w396:refnum<class "AnalogOutput.lvclass">)
          n160 = Bundle By Name(cluster=w412, "AnalogOutput"=w396, "2020Error"=w389) -> (w411:refnum<class "AtomChipHWC.lvclass">)
        }
        frame "HMP2030" {
          # "add configure for either voltage or current programming"
          n161 = Unbundle By Name(w447) -> ("AnalogOutput"=w438:refnum<class "AnalogOutput.lvclass">, "2030Error"=w426:errorcluster)
          n162 = Number To Decimal String(number=w429) -> (decimal integer string=w430:string)  [unwired: 1 in]
          n163 = call "getName.vi"("error in (no error)"=w440, "AnalogOutput.lvclass in"=w439) -> ("error out"=w445:errorcluster, "name"=w428:string, "AnalogOutput.lvclass out"=w443:refnum<class "AnalogOutput.lvclass">)  [unwired: 7 in]
          n164 = Concatenate Strings(w430, w428) -> (w427:string)
          n165 = call-dynamic "getPhysicalChannels.vi"("AnalogOutput.lvclass in"=w443, "error in (no error)"=w445) -> ("AnalogOutput.lvclass out"=w442:refnum<class "AnalogOutput.lvclass">, "Physical Channels"=w437:string, "error out"=w444:errorcluster)
          n166 = call "getRanges.vi"("AnalogOutput.lvclass in"=w442, "error in (no error)"=w444) -> ("AnalogOutput.lvclass out"=w441:refnum<class "AnalogOutput.lvclass">, "Ranges"=w436:dbl[], "error out"=w422:errorcluster)
          n167 = Bundle(w427, "Physical Channels"=w437, "Ranges"=w436) -> (w435:T1)  [unwired: 1 in]
          n168 = call "getTimingProperties.vi"("AnalogOutput.lvclass in"=w441, "error in (no error)"=w422) -> ("AnalogOutput.lvclass out"=w421:refnum<class "AnalogOutput.lvclass">, "Timing"=w434:T2, "error out"=w420:errorcluster)
          n169 = call-dynamic "configureForVoltageOutput.vi"("error in (no error)"=w426, "Output Properties"=w435, "AnalogOutput in"=w438) -> ("error out"=w425:errorcluster, "AnalogOutput out"=w433:refnum<class "AnalogOutput.lvclass">)
          n170 = call-dynamic "configureTiming.vi"("error in (no error)"=w425, "Timing"=w434, "AnalogOutput in"=w433) -> ("error out"=w416:errorcluster, "AnalogOutput out"=w417:refnum<class "AnalogOutput.lvclass">)
          n171 = call "getTimes.vi"("error in (no error)"=w420, "AnalogOutput in"=w421) -> ("error out"=w418:errorcluster, "times"=w413:dbl[], "AnalogOutput out"=w419:refnum<class "AnalogOutput.lvclass">)  [unwired: 7 in]
          n172 = call "setTimes.vi"("error in (no error)"=w416, "times"=w413, "AnalogOutput in"=w417) -> ("error out"=w415:errorcluster, "AnalogOutput out"=w414:refnum<class "AnalogOutput.lvclass">)  [unwired: 7 in]
          n173 = call "getData.vi"("error in (no error)"=w418, "AnalogOutput.lvclass in"=w419) -> ("error out"=w423:errorcluster, "Data"=w432:dbl[][])  [unwired: 7 in, 1 out]
          n174 = call-dynamic "loadData.vi"("error in (no error)"=w415, "Data"=w432, "AnalogOutput in"=w414) -> ("error out"=w424:errorcluster, "AnalogOutput out"=w431:refnum<class "AnalogOutput.lvclass">)
          n175 = Bundle By Name(cluster=w447, "AnalogOutput"=w431, "2030Error"=w424) -> (w446:refnum<class "AtomChipHWC.lvclass">)
        }
        frame "HMP4030" {
          # "add configure for either voltage or current programming"
          n176 = Unbundle By Name(w482) -> ("AnalogOutput"=w473:refnum<class "AnalogOutput.lvclass">, "4030Error"=w461:errorcluster)
          n177 = Number To Decimal String(number=w464) -> (decimal integer string=w465:string)  [unwired: 1 in]
          n178 = call "getName.vi"("error in (no error)"=w475, "AnalogOutput.lvclass in"=w474) -> ("error out"=w480:errorcluster, "name"=w463:string, "AnalogOutput.lvclass out"=w478:refnum<class "AnalogOutput.lvclass">)  [unwired: 7 in]
          n179 = Concatenate Strings(w465, w463) -> (w462:string)
          n180 = call-dynamic "getPhysicalChannels.vi"("AnalogOutput.lvclass in"=w478, "error in (no error)"=w480) -> ("AnalogOutput.lvclass out"=w477:refnum<class "AnalogOutput.lvclass">, "Physical Channels"=w472:string, "error out"=w479:errorcluster)
          n181 = call "getRanges.vi"("AnalogOutput.lvclass in"=w477, "error in (no error)"=w479) -> ("AnalogOutput.lvclass out"=w476:refnum<class "AnalogOutput.lvclass">, "Ranges"=w471:dbl[], "error out"=w457:errorcluster)
          n182 = Bundle(w462, "Physical Channels"=w472, "Ranges"=w471) -> (w470:T1)  [unwired: 1 in]
          n183 = call "getTimingProperties.vi"("AnalogOutput.lvclass in"=w476, "error in (no error)"=w457) -> ("AnalogOutput.lvclass out"=w456:refnum<class "AnalogOutput.lvclass">, "Timing"=w469:T2, "error out"=w455:errorcluster)
          n184 = call-dynamic "configureForVoltageOutput.vi"("error in (no error)"=w461, "Output Properties"=w470, "AnalogOutput in"=w473) -> ("error out"=w460:errorcluster, "AnalogOutput out"=w468:refnum<class "AnalogOutput.lvclass">)
          n185 = call-dynamic "configureTiming.vi"("error in (no error)"=w460, "Timing"=w469, "AnalogOutput in"=w468) -> ("error out"=w451:errorcluster, "AnalogOutput out"=w452:refnum<class "AnalogOutput.lvclass">)
          n186 = call "getTimes.vi"("error in (no error)"=w455, "AnalogOutput in"=w456) -> ("error out"=w453:errorcluster, "times"=w448:dbl[], "AnalogOutput out"=w454:refnum<class "AnalogOutput.lvclass">)  [unwired: 7 in]
          n187 = call "setTimes.vi"("error in (no error)"=w451, "times"=w448, "AnalogOutput in"=w452) -> ("error out"=w450:errorcluster, "AnalogOutput out"=w449:refnum<class "AnalogOutput.lvclass">)  [unwired: 7 in]
          n188 = call "getData.vi"("error in (no error)"=w453, "AnalogOutput.lvclass in"=w454) -> ("error out"=w458:errorcluster, "Data"=w467:dbl[][])  [unwired: 7 in, 1 out]
          n189 = call-dynamic "loadData.vi"("error in (no error)"=w450, "Data"=w467, "AnalogOutput in"=w449) -> ("error out"=w459:errorcluster, "AnalogOutput out"=w466:refnum<class "AnalogOutput.lvclass">)
          n190 = Bundle By Name(cluster=w482, "AnalogOutput"=w466, "4030Error"=w459) -> (w481:refnum<class "AtomChipHWC.lvclass">)
        }
      }
      n191 = call "addConfiguredDevice.vi"("error in (no error)"=w22, "deviceName"=w21, "HWController in"=w23) -> ("error out"=w10:errorcluster, "HWController out"=w12:refnum<class "AtomChipHWC.lvclass">)  [unwired: 7 in]
      n192 = case shown="True" w8 {
        tunnel: w12 -> [w26 w31]
        tunnel: [w26 w30] -> w11
        tunnel: w10 -> [w25 w29]
        tunnel: [w25 w28] -> w9
        frame False {
        }
        frame True {
          n193 = call-dynamic "removedConfiguredDevice.vi"("error in (no error)"=w29, "device"="Ao8b", "HWController in"=w31) -> ("error out"=w28:errorcluster, "HWController out"=w30:refnum<class "AtomChipHWC.lvclass">)  [unwired: 7 in]
        }
      }
    }
    frame Error {
    }
  }
  "error out" <- w6
  "AtomChipHWC out" <- w4
  n194 = Request Deallocation(TRUE) -> ()
